vi "CCM-XControl Data to Tables.vi"(0 "Channels By Device":cluster{"Out":string[], "In":string[]}[](array[cluster]), 7 "Endpoints by Channel by Device":cluster{"Outputs":string[], "Inputs":string[]}[](array[cluster])) -> (4 "Tables":cluster{"Table":T1[]}[](array[cluster]))   [LabVIEW 2020]
uses:
  Type Defs/CM-Connection.ctl
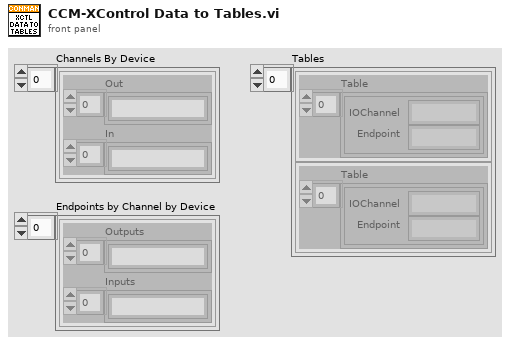
[diagram p1: front panel]
types:
  T1 = typedef "CM-Connection.ctl" = cluster{"IOChannel":string, "Endpoint":string}
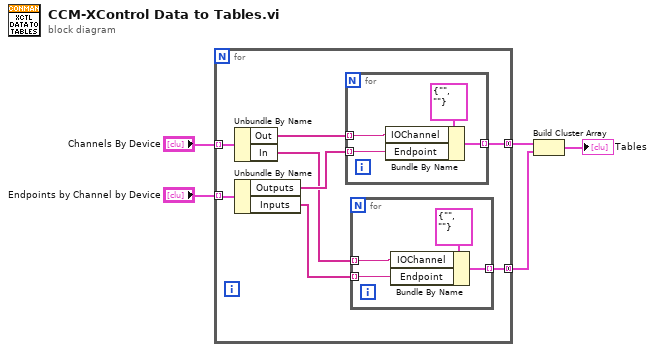
[diagram p0: block diagram]
diagram:
  n1 = for {
    tunnel: "Channels By Device" -> [w13] mode=indexing
    tunnel: "Endpoints by Channel by Device" -> [w12] mode=indexing
    tunnel: [w9] -> w3 mode=concatenating
    tunnel: [w6] -> w2 mode=concatenating
    n2 = Unbundle By Name(w13) -> ("Out"=w11:string[], "In"=w8:string[])
    n3 = Unbundle By Name(w12) -> ("Outputs"=w10:string[], "Inputs"=w7:string[])
    n4 = for {
      tunnel: w11 -> [w20] mode=indexing
      tunnel: w10 -> [w19] mode=indexing
      tunnel: [w18] -> w9 mode=indexing
      n5 = Bundle By Name(cluster=T1 {"IOChannel"="", "Endpoint"=""}, "IOChannel"=w20, "Endpoint"=w19) -> (w18:T1)
    }
    n6 = for {
      tunnel: w8 -> [w16] mode=indexing
      tunnel: w7 -> [w15] mode=indexing
      tunnel: [w14] -> w6 mode=indexing
      n7 = Bundle By Name(cluster=T1 {"IOChannel"="", "Endpoint"=""}, "IOChannel"=w16, "Endpoint"=w15) -> (w14:T1)
    }
  }
  n8 = Build Cluster Array(w3, w2) -> (→"Tables":cluster{T1[]}[])
